vi "SCI_Rx_Validate.vi"(0 "Head":u16=170 format="%x", 5 "Data8Hghr":u16 format="%x", 7 "Data8Lwr":u16 format="%x", 9 "Type":u16 format="%x", 11 "CrcRsd":u16 format="%x") -> (4 "SciPckOut":T1={"包头"=170, "数据低8位"=0, "数据低高8位"=0, "数据类型"=0, "CRC余数"=0, "数据无效"=FALSE, "数据更新"=FALSE} {"包头" format="%02x"; "数据低8位" format="%02x"; "数据低高8位" format="%02x"; "数据类型" items=["VOID"]; "CRC余数" format="%02x"})   [LabVIEW 2015]
uses:
  SCI_DataPck.ctl
  SCI_DataType.ctl
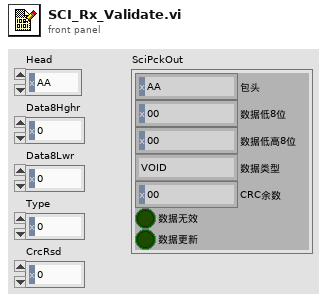
[diagram p1: front panel]
types:
  T1 = typedef "SCI_DataPck.ctl" = cluster{"包头":u16, "数据低8位":u16, "数据低高8位":u16, "数据类型":T2, "CRC余数":u16, "数据无效":bool, "数据更新":bool}
  T2 = typedef "SCI_DataType.ctl" = u16
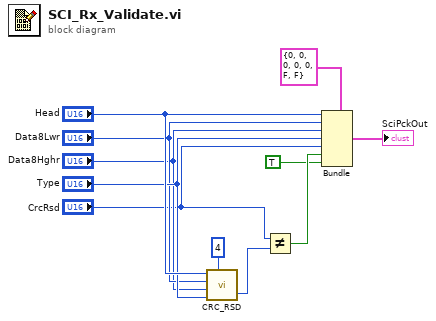
[diagram p0: block diagram]
diagram:
  n1 = call "CRC_RSD.vi"("BYTE 0"="Head", "BYTE 1"="Data8Lwr", "BYTE 2"="Data8Hghr", "BYTE 3"="Type", "Number of BYTE"=4) -> ("RSD"=w3:u16)
  n2 = Not Equal?(x="CrcRsd", y=w3) -> (x != y?=w2:bool)
  n3 = Bundle(cluster=T1 {"包头"=0, "数据低8位"=0, "数据低高8位"=0, "数据类型"=0, "CRC余数"=0, "数据无效"=FALSE, "数据更新"=FALSE} ("SciPckIn"), "包头"="Head", "数据低8位"="Data8Lwr", "数据低高8位"="Data8Hghr", "数据类型"="Type", "CRC余数"="CrcRsd", "数据无效"=w2, "数据更新"=TRUE) -> (→"SciPckOut":T1)
